vi "Phase current analysis.vi"() -> ()   [LabVIEW 2018]
uses:
  Stan.ctl
  <vilib>/express/express analysis/Spectral/Block/exnSpectralBlock spectral measurements power poly.vi
  <vilib>/express/express analysis/Spectral/Block/exnSpectralBlock spectral measurements power DDT.vi
  <vilib>/express/express analysis/Spectral/Block/exnSpectralBlock spectral measurements power WFM.vi
  <vilib>/Utility/file.llb/Write Delimited Spreadsheet (DBL).vi
  <vilib>/express/express analysis/Spectral/XNode/ExpressSpectralMeasurementsBlockNode.xnode
panel:
  out "Rzeczywste fp [Hz]":dbl[](array[numeric])
  out "A_fp [dbB]":dbl[](array[numeric])
  out "fp i 2fp":dbl[](array[numeric])
  out "FFT - I_p":cluster{"f0":dbl, "df":dbl, "magnitude":dbl[]}(graph) caption="Signals"
  out "XY Graph":cluster{"I_alfa":dbl[], "i_beta":dbl[]}(graph)
  out "Liczba prętów":dbl
  in  "Ścieżka do zapisu":path
  out "Obliczone A[dB]":dbl[](array[numeric])
  out "Rzeczywiste f [Hz]":dbl[](array[numeric])
  in  "Zakres poszukiwanych\n   częstotliwośći [Hz]":dbl=1.5
  out "fp -":dbl
  out "fp +":dbl
  out "Poślizg s":dbl
  out "Prędkość synchroniczna":dbl
  out "Częstotliwość zasilania f_s":dbl
  out "Prędkość zmierzona":dbl
  out "FFT fazy C":dynamicdata(graph) caption="Signals"
  in  "Tab Control":T1(tab)
  out "Faza A":dynamicdata(graph) caption="Signals"
  out "Faza B":dynamicdata(graph) caption="Signals"
  out "Faza C":dynamicdata(graph) caption="Signals"
  out "Prądy fazowe stojana":dynamicdata(graph) caption="Signals"
  in  "Analiza":bool
  in  "Zapis":bool
  in  "Stop":bool
  in  "Odczyt":bool
  # "Metoda wykorzystująca analizę widmową"
  # "Posiadane parametry"
  # "Parametry obliczone"
  # "Poszukiwane obszary widma"
  # "fs"
  # "fp +"
  # "fp -"
  # "Metoda wykorzystująca moduł wektora przestrzennego"
  # "fp"
  # "2fp"
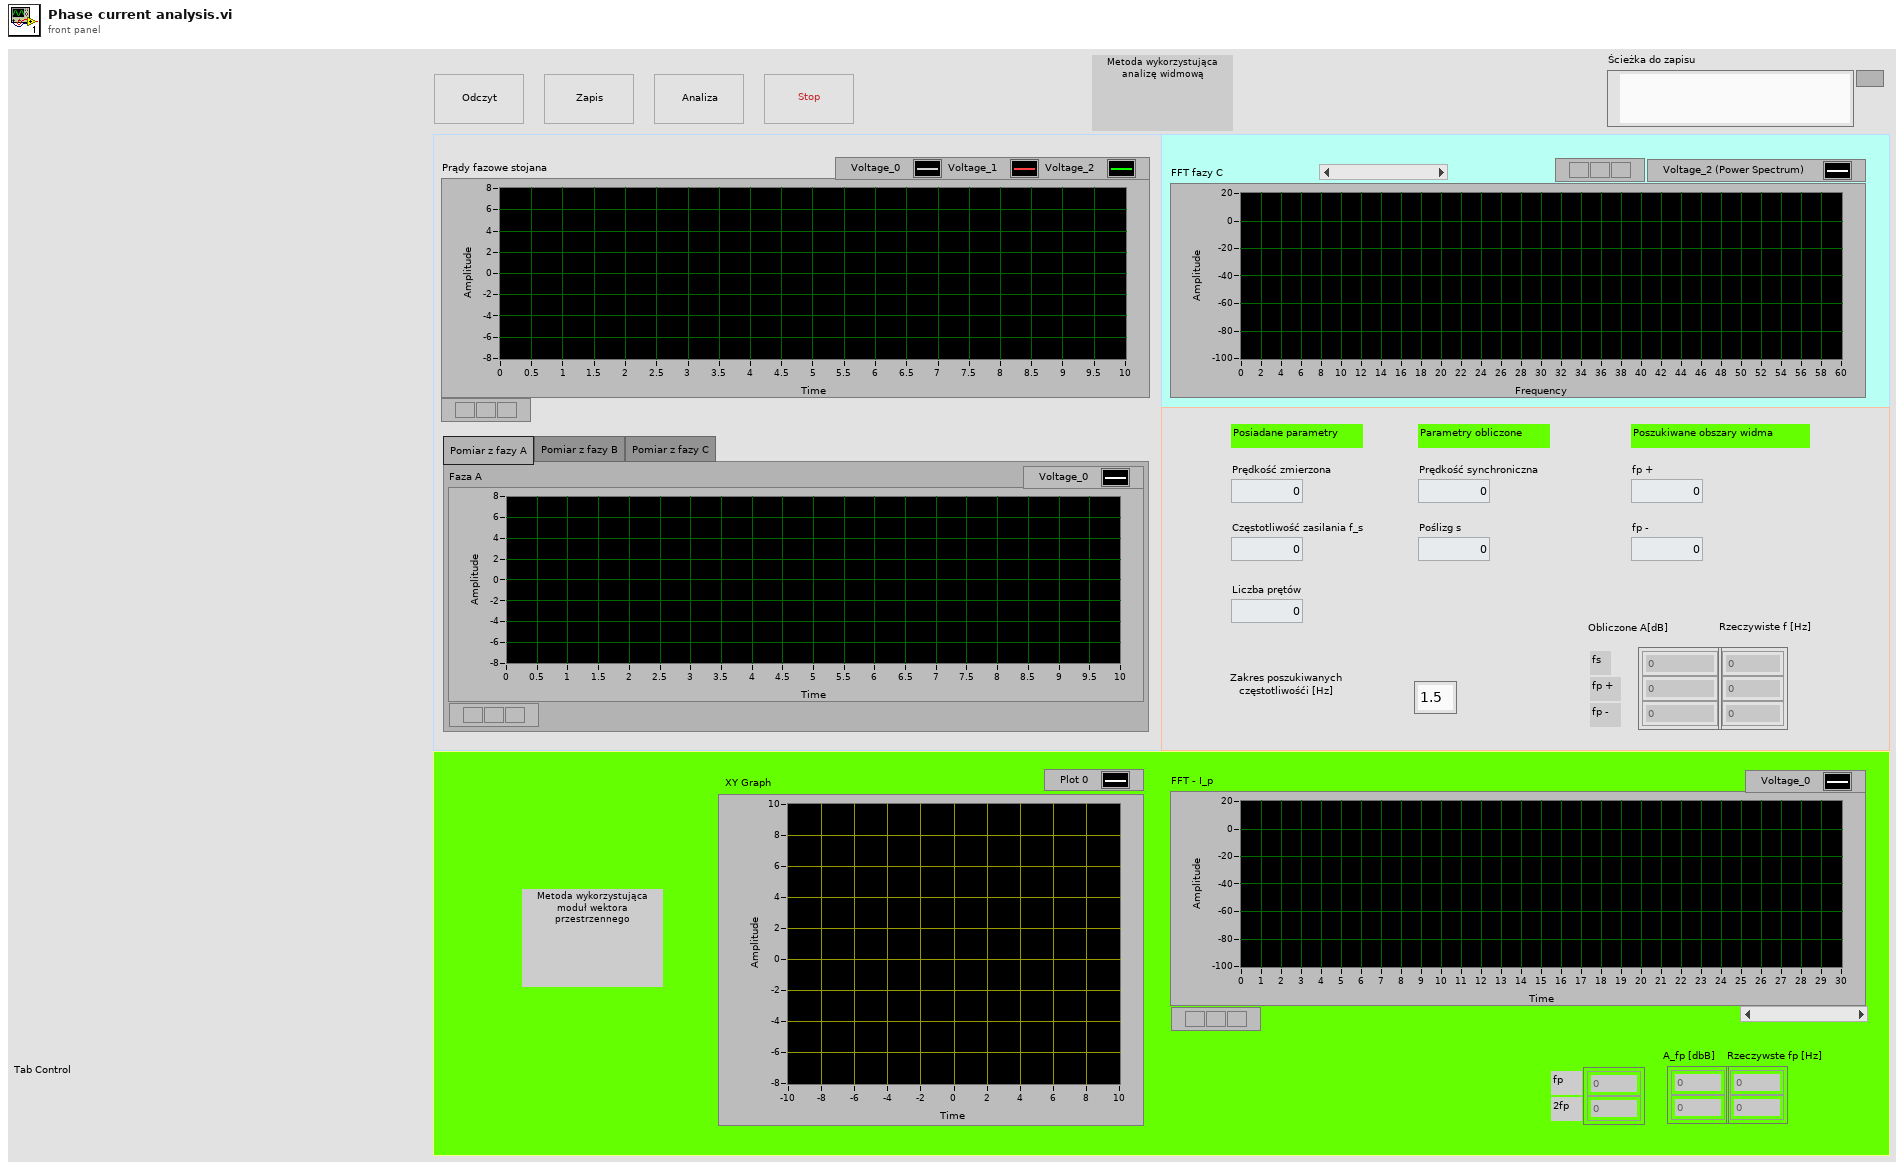
[diagram p1: front panel]
types:
  T1 = enum32{"Pomiar z fazy A", "Pomiar z fazy B", "Pomiar z fazy C"}
  T2 = typedef "Stan.ctl" = enum16{"Oczekiwanie", "Odczyt", "Analiza", "Analiza MWP", "Zapis", "Stop"}
  T3 = cluster{"averaging mode":u16, "weighting mode":u16, "number of averages":u32}
  T4 = cluster{"dB On (F)":bool, "unwrap phase (F)":bool, "convert to degree (F)":bool}
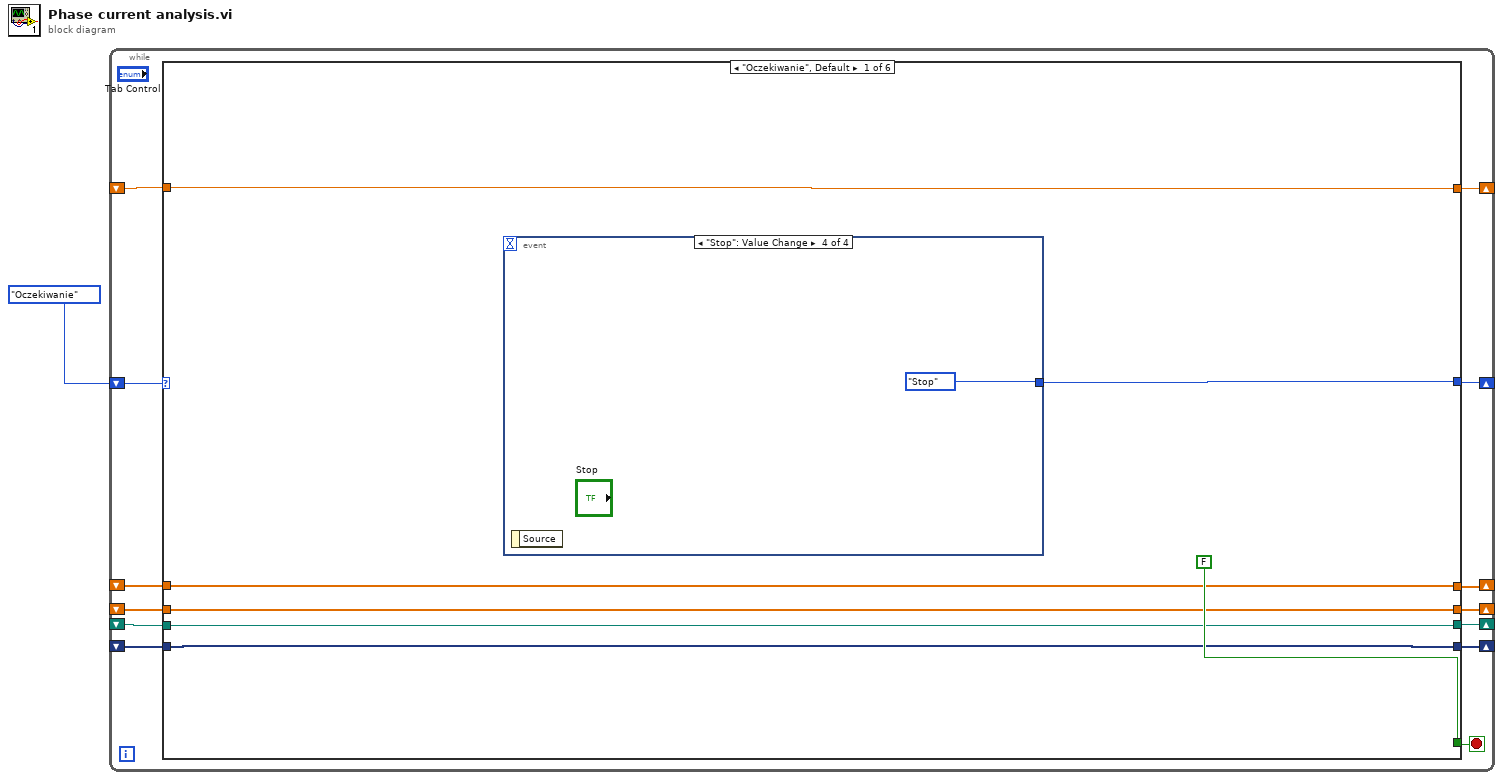
[diagram p0: block diagram]
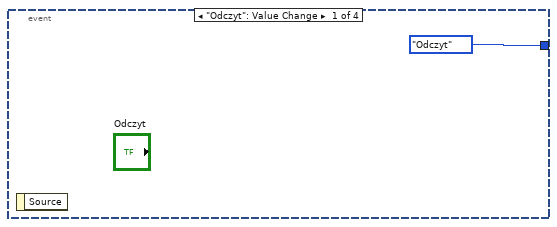
[diagram p2: hidden frame]
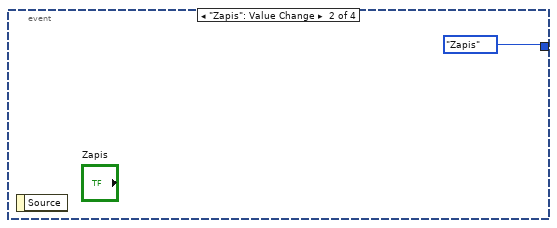
[diagram p3: hidden frame]
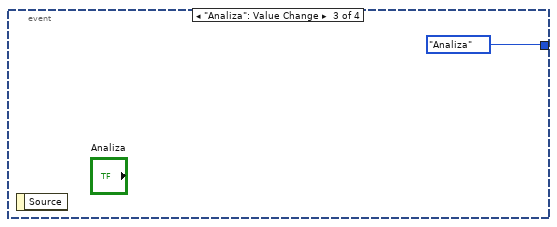
[diagram p4: hidden frame]
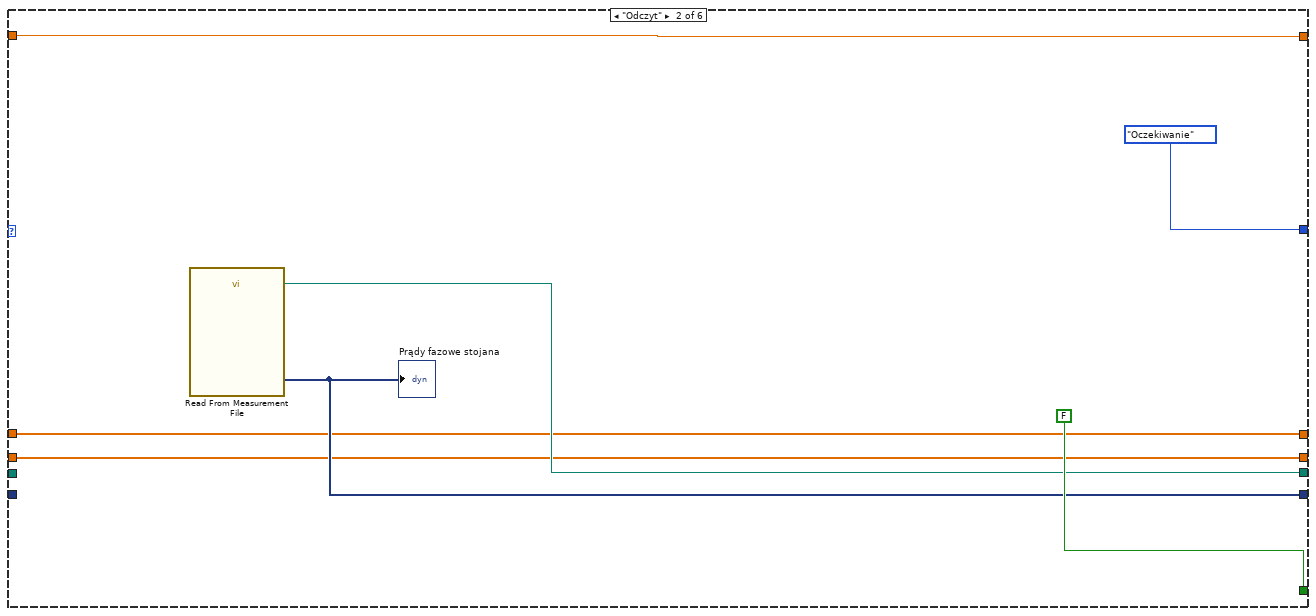
[diagram p5: hidden frame]
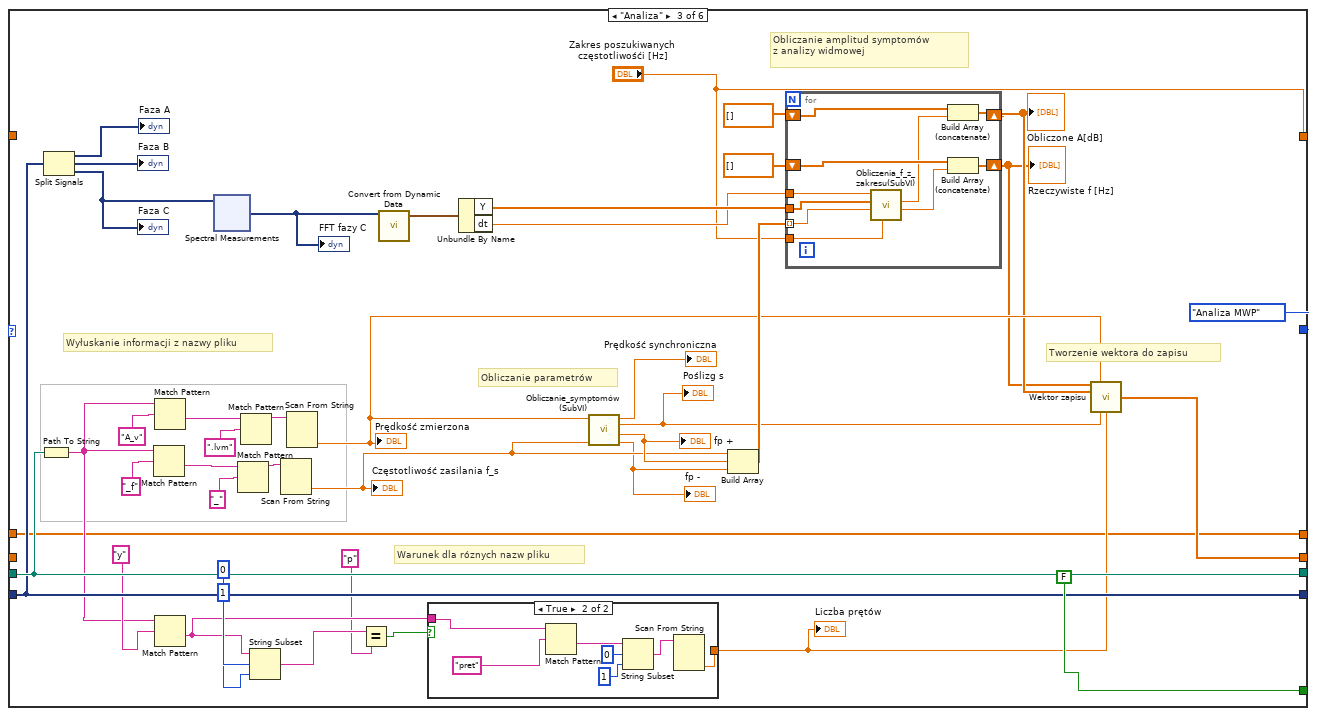
[diagram p6: hidden frame]
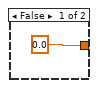
[diagram p7: hidden frame]
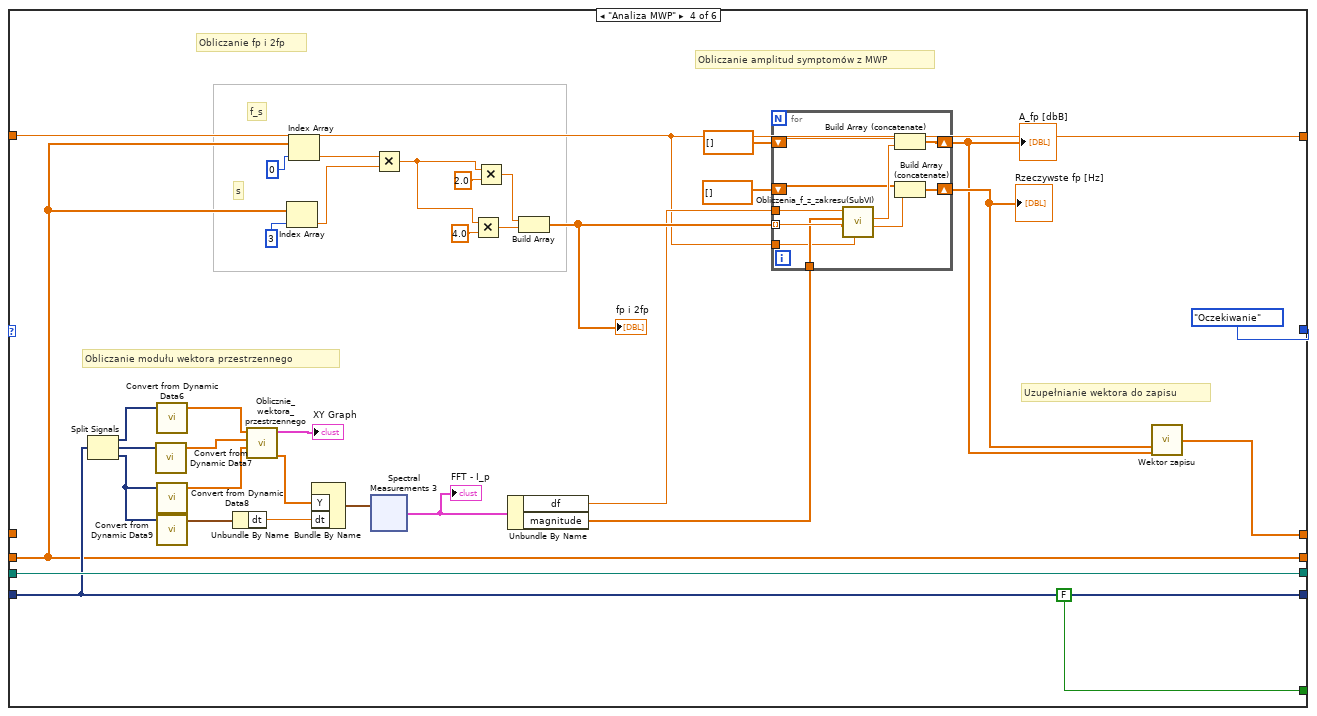
[diagram p8: hidden frame]
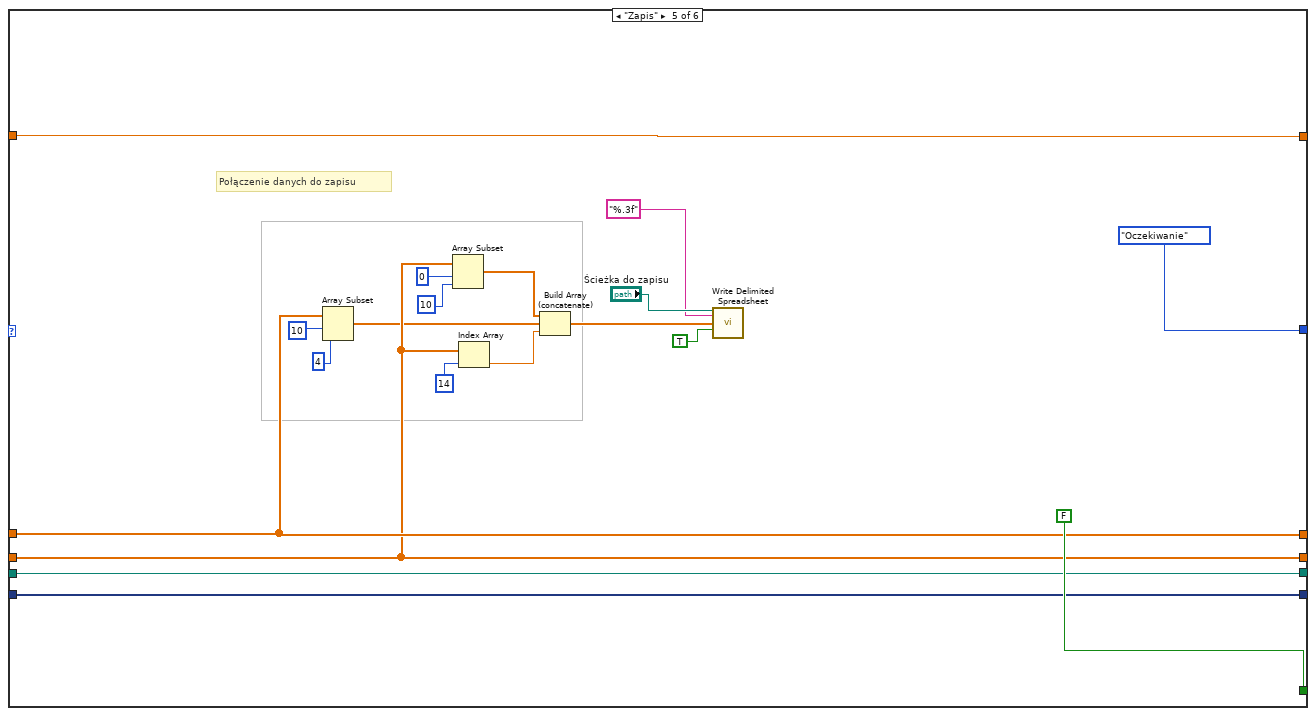
[diagram p9: hidden frame]
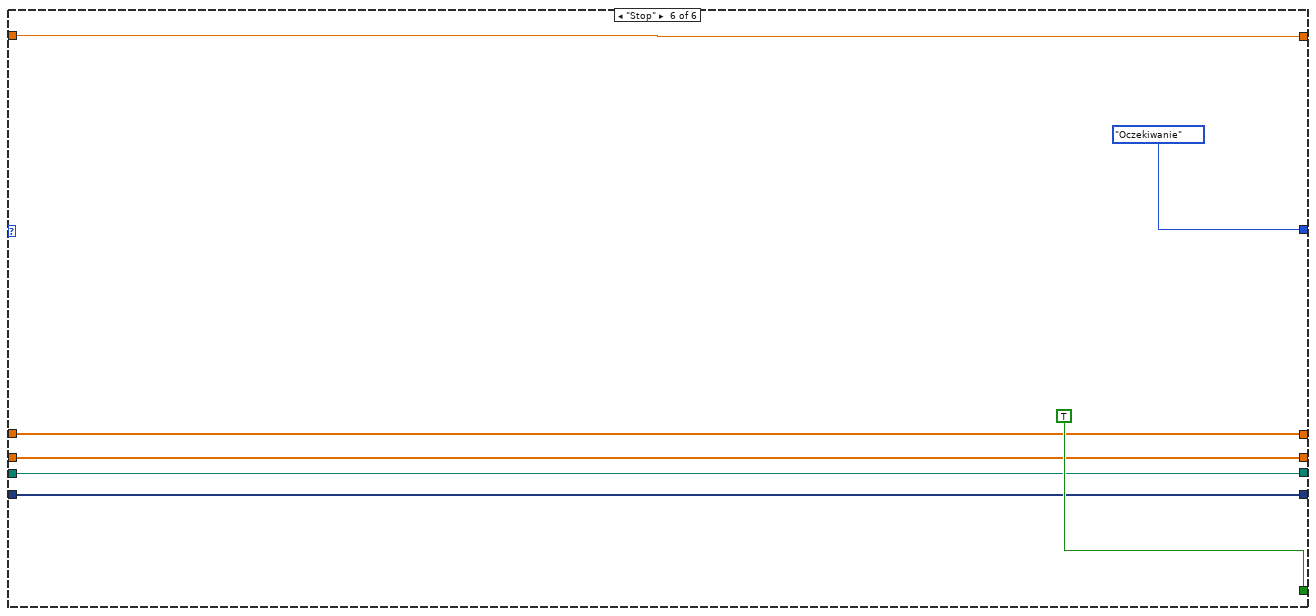
[diagram p10: hidden frame]
diagram:
  n1 = while {
    shift-right: [w13] -> _
    shift-left: Stan."Oczekiwanie" -> [w14]
    shift-right: [w11] -> _
    shift-left: _ -> [w8]
    shift-right: [w10] -> _
    shift-left: _ -> [w9]
    shift-right: [w7] -> _
    shift-left: _ -> [w6]
    shift-right: [w5] -> _
    shift-left: _ -> [w4]
    shift-right: [w3] -> _
    shift-left: _ -> [w2]
    stop <- w12 stop-if-true
    n2 = case shown="\"Oczekiwanie\", Default" w14 {
      tunnel: [w21 Stan."Oczekiwanie" Stan."Analiza MWP" Stan."Oczekiwanie" Stan."Oczekiwanie" Stan."Oczekiwanie"] -> w13
      tunnel: [FALSE FALSE FALSE FALSE FALSE TRUE] -> w12
      tunnel: [w18 w30 w63 w131 w171 w178] -> w11
      tunnel: [w19 w29 w64 w136 w172 w179] -> w10
      tunnel: w9 -> [w19 _ w64 w136 w172 w179]
      tunnel: w8 -> [w18 _ w63 w131 w171 w178]
      tunnel: [w17 w28 w39 w104 w162 w177] -> w7
      tunnel: w6 -> [w17 w28 _ w104 w162 w177]
      tunnel: [w16 w27 "Zakres poszukiwanych\n   częstotliwośći [Hz]" w111 w168 w176] -> w5
      tunnel: w4 -> [w16 w27 _ w111 w168 w176]
      tunnel: [w15 w26 w33 w102 w167 w175] -> w3
      tunnel: w2 -> [w15 w26 w33 _ w167 w175]
      frame "Oczekiwanie", Default {
        n3 = event shown="[3] \"Stop\": Value Change" {
          selector: _ -> [_ _ _ _]
          dyn-events: _ -> [_ _ _ _]
          timeout: _ -> [_ _ _ _]
          tunnel: [Stan."Odczyt" Stan."Zapis" Stan."Analiza" Stan."Stop"] -> w21
          event "Odczyt": Value Change {
            n4 = event-data() -> ()  [unwired: 1 in, 1 out]
          }
          event "Zapis": Value Change {
            n5 = event-data() -> ()  [unwired: 1 in, 1 out]
          }
          event "Analiza": Value Change {
            n6 = event-data() -> ()  [unwired: 1 in, 1 out]
          }
          event "Stop": Value Change {
            n7 = event-data() -> ()  [unwired: 1 in, 1 out]
          }
        }
      }
      frame "Odczyt" {
        n8 = call "Read From Measurement File"() -> ("Filename Out"=w29:path, "Signals"=w30:dynamicdata)  [unwired: 6 in, 4 out]
        "Prądy fazowe stojana" <- w30
      }
      frame "Analiza" {
        # "Wyłuskanie informacji z nazwy pliku"
        # "Warunek dla róznych nazw pliku"
        # "Tworzenie wektora do zapisu"
        # "Obliczanie parametrów"
        # "Obliczanie amplitud symptomów \nz analizy widmowej"
        n9 = Path To String(path=w64) -> (string=w47:string)
        n10 = Split Signals(w63) -> (→"Faza A":dynamicdata, →"Faza B":dynamicdata, w51:dynamicdata)  [unwired: 3 in]
        "Faza C" <- w51
        n11 = Match Pattern(string=w47, regular expression="_f") -> (after substring=w67:string)  [unwired: 1 in, 3 out]
        n12 = Match Pattern(string=w47, regular expression="A_v") -> (after substring=w71:string)  [unwired: 1 in, 3 out]
        n13 = Match Pattern(string=w47, regular expression="y") -> (after substring=w44:string)  [unwired: 1 in, 3 out]
        n14 = xnode ("Spectral Measurements")("Signals"=w51) -> ("Power Spectrum"=w62:dynamicdata)  [unwired: 1 in, 1 out]
        "FFT fazy C" <- w62
        n15 = Match Pattern(string=w67, regular expression="_") -> (before substring=w66:string)  [unwired: 1 in, 3 out]
        n16 = Match Pattern(string=w71, regular expression=".lvm") -> (before substring=w69:string)  [unwired: 1 in, 3 out]
        n17 = String Subset(string=w44, offset (0)=0, length (rest)=1 ("length (rest)")) -> (substring=w43:string)
        n18 = Scan From String(input string=w66) -> (output 1=w50:dbl)  [unwired: 4 in, 3 out]
        "Częstotliwość zasilania f_s" <- w50
        n19 = Scan From String(input string=w69) -> (output 1=w38:dbl)  [unwired: 4 in, 3 out]
        "Prędkość zmierzona" <- w38
        n20 = Equal?(x=w43, y="p") -> (x = y?=w41:bool)
        n21 = call "Convert from Dynamic Data"("Dynamic Data Type"=w62) -> ("Waveform"=w57:waveform(dbl))  [unwired: 3 in]
        n22 = case shown="True" w41 {
          tunnel: [0.0 w77] -> w34
          tunnel: w44 -> [_ w76]
          frame False {
          }
          frame True {
            n23 = Match Pattern(string=w76, regular expression="pret") -> (after substring=w82:string)  [unwired: 1 in, 3 out]
            n24 = String Subset(string=w82, offset (0)=0, length (rest)=1 ("length (rest)")) -> (substring=w78:string)
            n25 = Scan From String(input string=w78) -> (output 1=w77:dbl)  [unwired: 4 in, 3 out]
          }
        }
        "Liczba prętów" <- w34
        n26 = Unbundle By Name ("Get Waveform Components")(w57) -> ("Y"=w58:dbl[], "dt"=w52:dbl)
        n27 = call "Obliczanie_symptomów (SubVI).vi"("V [obr/min]"=w38, "fs [Hz]"=w50) -> ("Prędkość synchroniczna"=→"Prędkość synchroniczna":dbl, "Poślizg"=w40:dbl, "fp +"=w56:dbl, "fp -"=w49:dbl)  [unwired: 5 in]
        "Poślizg s" <- w40
        "fp +" <- w56
        "fp -" <- w49
        n28 = Build Array(w50, w56, w49) -> (w55:dbl[])
        n29 = for {
          shift-right: [w92] -> w37
          shift-left: dbl[] [] -> [w87]
          shift-right: [w91] -> w36
          shift-left: dbl[] [] -> [w89]
          tunnel: w55 -> [w86] mode=indexing
          tunnel: w52 -> [w85]
          tunnel: w58 -> [w84]
          tunnel: "Zakres poszukiwanych\n   częstotliwośći [Hz]" -> [w83]
          n30 = call "Obliczenia_f_z_zakresu(SubVI).vi"("Zakres"=w83, "Szukana częstotliwość"=w86, "magnitude"=w84, "df"=w85) -> ("częstotliwość szukanej f"=w90:dbl, "amplituda szukanej f"=w88:dbl)  [unwired: 5 in, 1 out]
          n31 = Build Array (concatenate)(w87, w88) -> (w92:dbl[])
          n32 = Build Array (concatenate)(w89, w90) -> (w91:dbl[])
        }
        "Rzeczywiste f [Hz]" <- w36
        "Obliczone A[dB]" <- w37
        n33 = call "Wektor zapisu.vi"("Rzeczywiste f [Hz]"=w36, "Prędkość zmierzona"=w38, "Obliczone Amplitudy[dB]"=w37, "Poślizg"=w40, "Liczba prętów"=w34) -> ("Wyjście"=w39:dbl[])  [unwired: 10 in]
      }
      frame "Analiza MWP" {
        # "s"
        # "f_s"
        # "Obliczanie fp i 2fp"
        # "Uzupełnianie wektora do zapisu"
        # "Obliczanie amplitud symptomów z MWP"
        # "Obliczanie modułu wektora przestrzennego"
        n34 = Split Signals(w131) -> (w133:dynamicdata, w132:dynamicdata, w127:dynamicdata)  [unwired: 3 in]
        n35 = call "Convert from Dynamic Data7"("Dynamic Data Type"=w132) -> ("Array"=w128:dbl[])  [unwired: 3 in]
        n36 = call "Convert from Dynamic Data6"("Dynamic Data Type"=w133) -> ("Array"=w130:dbl[])  [unwired: 3 in]
        n37 = call "Convert from Dynamic Data8"("Dynamic Data Type"=w127) -> ("Array"=w129:dbl[])  [unwired: 3 in]
        n38 = call "Convert from Dynamic Data9"("Dynamic Data Type"=w127) -> ("Waveform"=w126:waveform(dbl))  [unwired: 3 in]
        n39 = Unbundle By Name ("Get Waveform Components")(w126) -> ("dt"=w124:dbl)
        n40 = call "Oblicznie_wektora_przestrzennego.vi"("I_C"=w129, "I_B"=w128, "I_A"=w130) -> ("i_p"=w123:dbl[], "i_alfa, i_beta"=→"XY Graph":cluster{dbl[], dbl[]})  [unwired: 7 in]
        n41 = Index Array(array=w104, index=3) -> (element=w105:dbl)
        n42 = Index Array(array=w104, index=0) -> (element=w107:dbl)
        n43 = Bundle By Name("Y"=w123, "dt"=w124) -> (w125:waveform(dbl))  [unwired: 1 in]
        n44 = xnode ("Spectral Measurements 3")("Signals"=w125) -> ("Power Spectrum"=w121:cluster{"f0":dbl, "df":dbl, "magnitude":dbl[]})  [unwired: 1 in, 1 out]
        "FFT - I_p" <- w121
        n45 = Multiply(x=w107, y=w105) -> (x*y=w103:dbl)
        n46 = Multiply(x=w103, y=4.0) -> (x*y=w118:dbl)
        n47 = Multiply(x=w103, y=2.0) -> (x*y=w117:dbl)
        n48 = Unbundle By Name(w121) -> ("df"=w113:dbl, "magnitude"=w112:dbl[])
        n49 = Build Array(w117, w118) -> (w114:dbl[])
        "fp i 2fp" <- w114
        n50 = for {
          shift-right: [w145] -> w109
          shift-left: dbl[] [] -> [w144]
          shift-right: [w143] -> w110
          shift-left: dbl[] [] -> [w141]
          tunnel: w114 -> [w140] mode=indexing
          tunnel: w113 -> [w139]
          tunnel: w112 -> [w138]
          tunnel: w111 -> [w137]
          n51 = call "Obliczenia_f_z_zakresu(SubVI).vi"("Zakres"=w137, "Szukana częstotliwość"=w140, "magnitude"=w138, "df"=w139) -> ("częstotliwość szukanej f"=w142:dbl, "amplituda szukanej f"=w146:dbl)  [unwired: 5 in, 1 out]
          n52 = Build Array (concatenate)(w144, w146) -> (w145:dbl[])
          n53 = Build Array (concatenate)(w141, w142) -> (w143:dbl[])
        }
        "A_fp [dbB]" <- w109
        "Rzeczywste fp [Hz]" <- w110
        n54 = call "Wektor zapisu.vi"("Rzeczywiste fp [Hz]"=w110, "Obliczone Amplitudy_fp [dB]"=w109) -> ("Wyjście"=w102:dbl[])  [unwired: 13 in]
      }
      frame "Zapis" {
        # "Połączenie danych do zapisu"
        n55 = Array Subset(array=w167, index=10, length=4) -> (w159:dbl[])
        n56 = Array Subset(array=w162, index=0, length=10) -> (w160:dbl[])
        n57 = Index Array(array=w162, index=14) -> (element=w158:dbl)
        n58 = Build Array (concatenate)(w160, w159, w158) -> (w157:dbl[])
        n59 = call-poly <vilib>:"Write Delimited Spreadsheet.vi"("file path (dialog if empty)"="Ścieżka do zapisu", "format (%.3f)"="%.3f", "1D data"=w157, "append to file? (new file:F)"=TRUE) -> ()  [unwired: 10 in, 2 out]
      }
      frame "Stop" {
      }
    }
  }
